vi "ToDigital.vi"(8 "error in":errorcluster, 11 "Generic in":refnum<class "Generic.lvclass">) -> (0 "error out":errorcluster, 3 "Control out":refnum<class "Digital.lvclass">)   [LabVIEW 2014, in "Digital.lvclass"]
uses:
  Digital.lvclass
  Generic/Generic.lvclass
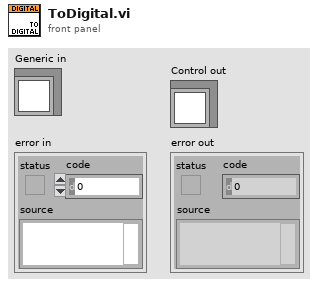
[diagram p1: front panel]
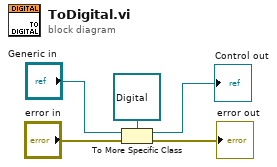
[diagram p0: block diagram]
diagram:
  n1 = To More Specific Class(target class=refnum<class "Digital.lvclass"> refnum ("Tab out"), reference="Generic in", error in="error in") -> (specific class reference=→"Control out":refnum<class "Digital.lvclass">, error out=→"error out":errorcluster)
